vi "Config Comparator Harmonics.vi"(0 "VISA resource name":refnum<visa-resource-name>, 1 "Element (1: Element 1)":u16(ring)=1 items=["", "Element1", "Element2", "Element3", "Sigma"], 5 "Channel (1)":u16=1 min=1 max=4 step=1, 7 "Harmo Limit Item (2: V)":u16(ring)=2 items=["OFF", "VTHD", "V", "VCON", "ATHD", "A", "ACON", "PF", "W", "WCON", "Vdeg", "Adeg"], 9 "Harmo Limit Value (0)":dbl min=-9999000000.0 max=9999000000.0 format="%^.3e", 11 "error in (no error)":errorcluster, 12 "Order (1)":u16=1 min=1 max=50 step=1) -> (4 "VISA resource name out":refnum<visa-resource-name>, 15 "error out":errorcluster)   [LabVIEW 2013, in "Yokogawa WT200 Series.lvlib"]
doc: "This VI sends the comparator limit values commands of harmonics measurement to the WT200 Series.\n\nNote : It needs /CMP and /HRM options."
uses:
  <instrlib>/Yokogawa WT200 Series/Yokogawa WT200 Series.lvlib
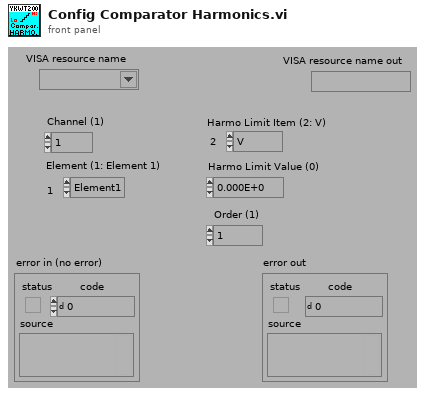
[diagram p1: front panel]
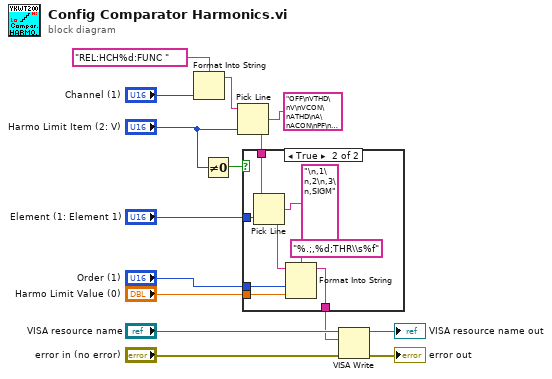
[diagram p0: block diagram]
diagram:
  n1 = Format Into String(format string="REL:HCH%d:FUNC ", "Channel (1)") -> (resulting string=w10:string)  [unwired: 2 in, 1 out]
  n2 = Not Equal To 0?(x="Harmo Limit Item (2: V)") -> (x != 0?=w4:bool)
  n3 = Pick Line(string ("")=w10, multi-line string="OFF\nVTHD\nV\nVCON\nATHD\nA\nACON\nPF\nW\nWCON\nVDEG\nADEG", line index="Harmo Limit Item (2: V)") -> (output string=w5:string)
  n4 = case shown="True" w4 {
    tunnel: w5 -> [w16 w19]
    tunnel: [w16 w24] -> w6
    tunnel: "Harmo Limit Value (0)" -> [_ w23]
    tunnel: "Order (1)" -> [_ w22]
    tunnel: "Element (1: Element 1)" -> [_ w17]
    frame False {
      # "OFF"
    }
    frame True {
      n5 = Pick Line(string ("")=w19, multi-line string="\n,1\n,2\n,3\n,SIGM" ("ÏÙÁ×²Ý•¶Žš—ñ"), line index=w17) -> (output string=w18:string)
      n6 = Format Into String(format string="%.;,%d;THR\\s%f", initial string=w18, w22, w23) -> (resulting string=w24:string)  [unwired: 1 in, 1 out]
    }
  }
  n7 = VISA Write(VISA resource name="VISA resource name", write buffer=w6, error in (no error)="error in (no error)") -> (VISA resource name out=→"VISA resource name out":refnum<visa-resource-name>, error out=→"error out":errorcluster)  [unwired: 1 out]
